vi "ATV Program Global Variables.vi"() -> ()   [LabVIEW 2011]
panel:
  in  "Webcam Data":T1={"Clamp Settings"={"Contrast"=100, "Filter width"=100, "Steepness"=2, "Subsampling Ratio"=1, "Show Search Area"=FALSE, "Show Search Lines"=FALSE, "Show Edges Found"=FALSE, "Show Result"=FALSE}, "Color Plane"=0, "BCG"={"Brightness"=171.0, "Contrast"=55.999992, "Gamma"=2.0}} {"BCG"."Gamma" min=0.1 max=10 step=0.01 scale=10.0..0.1 scale format="%.1f"; "BCG"."Contrast" min=1 max=89 step=0.1 scale=30.0..60.0 scale format="%.2f"; "BCG"."Brightness" min=0 max=255 step=1 scale=0.0..255.0 scale format="%.2f"; "Color Plane" items=["Red", "Green", "Blue", "Hue", "Saturation", "Luminance", "Value", "Intensity"]}
  out "ATV Vision":T2(plugin-control)
  out "Logfile Graph":cluster{dbl[], dbl[]}[](graph)=[{[-121.82428, -121.82428, -121.82428, -121.82428, -121.82428, -121.82428, -121.82428, -121.82428, -121.82428, -121.82428, -121.82428, -121.82428, -121.82428, -121.82428, -121.82428, -121.82428, -121.82428, -121.82428, -121.82428, -121.82428, -121.82428, -121.82428, -121.82428, -121.82428, -121.82428, -121.82428, -121.82428, -121.82428, -121.82428, -121.82428, -121.82428, -121.82428, -121.82428, -121.82428, -121.82428, -121.82428, -121.82428, -121.82428, -121.82428, -121.82428, -121.82428, -121.82428, -121.82428, -121.82428, -121.82428, -121.82428, -121.82428, -121.82428, -121.82428, -121.82428, -121.82428, -121.82428, -121.824573, -121.824573, -121.824573, -121.824573, -121.824573, -121.824573, -121.824573, -121.824573, -121.824573, -121.824573, -121.824573, -121.824573, -121.824573, -121.824573, -121.824573, -121.824573, -121.824573, -121.824573, -121.824573, -121.824573, -121.824573, -121.824573, -121.824573, -121.824573, -121.824573, -121.824573, -121.824573, -121.824573, -121.824573, -121.824573, -121.824573, -121.824573, -121.824573, -121.824573, -121.824573, -121.824573, -121.824573, -121.824573, -121.824573, -121.824573, -121.824573, -121.824573, -121.824573, -121.824573, -121.824573, -121.824573, -121.824573, -121.824573, -121.824573, -121.824573, -121.824573, -121.824573, -121.824573, -121.824573, -121.824573, -121.824573, -121.824573, -121.824573, -121.824573, -121.824573, -121.824573, -121.824573, -121.824573, -121.824573, -121.824573, -121.824573, -121.824573, -121.824573, -121.824573, -121.824573, -121.824573, -121.824573, -121.824573, -121.824573, -121.824573, -121.824573, -121.824573, -121.824373, -121.824373, -121.824373, -121.824373, -121.824373, -121.824373, -121.824373, -121.824373, -121.824373, -121.824373, -121.824373, -121.824373, -121.824373, -121.824373, -121.824373, -121.824373, -121.824373, -121.824373, -121.824373, -121.824373, -121.824373, -121.824373, -121.824373, -121.824373, -121.824373, -121.824373], [39.690327, 39.690327, 39.690327, 39.690327, 39.690327, 39.690327, 39.690327, 39.690327, 39.690327, 39.690327, 39.690327, 39.690327, 39.690327, 39.690327, 39.690327, 39.690327, 39.690327, 39.690327, 39.690327, 39.690327, 39.690327, 39.690327, 39.690327, 39.690327, 39.690327, 39.690327, 39.690327, 39.690327, 39.690327, 39.690327, 39.690327, 39.690327, 39.690327, 39.690327, 39.690327, 39.690327, 39.690327, 39.690327, 39.690327, 39.690327, 39.690327, 39.690327, 39.690327, 39.690327, 39.690327, 39.690327, 39.690327, 39.690327, 39.690327, 39.69047, 39.69047, 39.69047, 39.69047, 39.69047, 39.69047, 39.69047, 39.69047, 39.69047, 39.69047, 39.69047, 39.69047, 39.69047, 39.69047, 39.69047, 39.69047, 39.69047, 39.69047, 39.69047, 39.69047, 39.69047, 39.69047, 39.69047, 39.69047, 39.69047, 39.69047, 39.69047, 39.69047, 39.69047, 39.69047, 39.69047, 39.69047, 39.69047, 39.69047, 39.69047, 39.69047, 39.69047, 39.69047, 39.69047, 39.69047, 39.69047, 39.69047, 39.69047, 39.69047, 39.69047, 39.69047, 39.69047, 39.69047, 39.69047, 39.69047, 39.69047, 39.69047, 39.69047, 39.69047, 39.69047, 39.69047, 39.69047, 39.6908, 39.6908, 39.6908, 39.6908, 39.6908, 39.6908, 39.6908, 39.6908, 39.6908, 39.6908, 39.6908, 39.6908, 39.6908, 39.6908, 39.6908, 39.6908, 39.6908, 39.6908, 39.6908, 39.6908, 39.6908, 39.6908, 39.6908, 39.6908, 39.6908, 39.6908, 39.6908, 39.6908, 39.6908, 39.6908, 39.6908, 39.6905, 39.6905, 39.6905, 39.6905, 39.6905, 39.6905, 39.6905, 39.6905, 39.6905, 39.6905, 39.6905, 39.6905, 39.6905, 39.6905, 39.6905, 39.6905, 39.6905, 39.6905]}, {[-121.824573, -121.824573, -121.824373, -121.824373, -121.824173, -121.824173], [39.69047, 39.6908, 39.6908, 39.6905, 39.6905, 39.69095]}, {[-121.82428, -121.82428, -121.82428, -121.82428, -121.82428, -121.82428, -121.82428, -121.82428, -121.82428, -121.82428, -121.82428, -121.82428, -121.82428, -121.82428, -121.82428, -121.82428, -121.82428, -121.82428, -121.82428, -121.82428, -121.82428, -121.82428, -121.82428, -121.82428, -121.82428, -121.82428, -121.82428, -121.82428, -121.82428, -121.82428, -121.82428, -121.82428, -121.82428, -121.82428, -121.82428, -121.82428, -121.82428, -121.82428, -121.824573, -121.824573, -121.824573, -121.824573, -121.824573, -121.824573, -121.824573, -121.824573, -121.824573, -121.824573, -121.824573, -121.824573, -121.824573, -121.824373, -121.824373, -121.824373, -121.824373, -121.824373, -121.824373, -121.824373, -121.824373, -121.824373, -121.824373, -121.824373, -121.824373, -121.824373, -121.824373, -121.824373, -121.824373, -121.824373, -121.824373, -121.824373, -121.824373, -121.824373, -121.824373, -121.824373, -121.824373, -121.824373, -121.824373], [39.690327, 39.690327, 39.690327, 39.690327, 39.690327, 39.690327, 39.690327, 39.690327, 39.690327, 39.690327, 39.690327, 39.690327, 39.690327, 39.690327, 39.690327, 39.690327, 39.690327, 39.690327, 39.690327, 39.690327, 39.690327, 39.690327, 39.690327, 39.690327, 39.690327, 39.690327, 39.690327, 39.690327, 39.690327, 39.690327, 39.690327, 39.690327, 39.690327, 39.690327, 39.690327, 39.690327, 39.690327, 39.690327, 39.6908, 39.6908, 39.6908, 39.6908, 39.6908, 39.6908, 39.6908, 39.6908, 39.6908, 39.6908, 39.6908, 39.6908, 39.6908, 39.6908, 39.6908, 39.6908, 39.6908, 39.6908, 39.6908, 39.6908, 39.6908, 39.6905, 39.6905, 39.6905, 39.6905, 39.6905, 39.6905, 39.6905, 39.6905, 39.6905, 39.6905, 39.6905, 39.6905, 39.6905, 39.6905, 39.6905, 39.6905, 39.6905, 39.6905]}]
  in  "Map":refnum<k7>(container)
  in  "Map Data":T3={"X"=1000.0, "Y"=1000.0, "Zoom"=19.0, "Map Type"="hybrid", "Google Maps API Key"="AIzaSyDQES5BW68QG5HzTQIG5gxZIUTr_OVHJhg", "Map Refresh Rate (ms)"=5000, "Navigation Path Color"=16860, "Navigation Path Weight"=3, "URL"="http://maps.googleapis.com/maps/api/staticmap?&zoom=13&size=1000x1000&maptype=roadmap&markers=color:blue%7Clabel:S%7C40.702147,-74.015794&markers=color:green%7Clabel:G%7C40.711614,-74.012318&markers=color:red%7Ccolor:red%7Clabel:C%7C40.718217,-73.998284&sensor=false", "Boundary Coordinates"=[{"Latitude"=39.690655, "Longitude"=-121.82408}, {"Latitude"=39.690815, "Longitude"=-121.823863}, {"Latitude"=39.691022, "Longitude"=-121.824048}, {"Latitude"=39.690845, "Longitude"=-121.824595}, {"Latitude"=39.690771, "Longitude"=-121.824607}, {"Latitude"=39.690668, "Longitude"=-121.824669}, {"Latitude"=39.69033, "Longitude"=-121.824234}, {"Latitude"=39.690448, "Longitude"=-121.824055}], "GPS Balloon Character"="1", "Boundary Path Color"=16774656, "Boundary Path Weight"=5, "GPS Balloon Size"="mid", "GPS Balloon Color"="blue", "GPS Path Color"=16711680, "GPS Path Weight"=1, "Disable Google Maps"=FALSE} {"Boundary Coordinates"."Longitude" format="%_12g"; "Boundary Coordinates"."Latitude" format="%_11g"; "Zoom" format="%#.1g"}
  in  "Arduino 2 Data":T4={"Arduino 2 VISA resource"="COM4", "Front Center I2C Data"=[], "Disable Arduino 2"=FALSE, "Rear Left I2C Data"=[], "Rear Right I2C Data"=[]} {"Rear Right I2C Data" format="%x"; "Rear Left I2C Data" format="%x"; "Front Center I2C Data" format="%x"}
  in  "RUN":bool
  in  "Arduino 1 Data":T5={"Arduino 1 VISA resource"="COM6", "Front Right Sonar Analog In Voltage"=5.0, "Front Left Sonar Analog In Voltage"=5.0, "Disable Arduino 1"=FALSE}
  in  "Sonar Data":T6={"Front Left Distance"=0.0, "Front Right Distance"=0.0, "Analog In Filter Rank"=10, "Front Center Distance"=0.0, "Rear Left Distance"=0.0, "Rear Right Distance"=0.0, "Front Left Threshold"=300.0, "Front Right Threshold"=300.0, "Front Center Threshold"=300.0, "Rear Left Threshold"=0.0, "Rear Right Threshold"=0.0}
  in  "Compass Data":cluster{"Angle Uncertainty":dbl, "Heading":dbl}={"Angle Uncertainty"=5.0, "Heading"=0.0}
  in  "Obstacle Avoidance Data":T7={"Obstacle Detected"=FALSE, "Drive Speed"="1", "Steer Angle"="500000", "Left Object"=FALSE, "Right Object"=FALSE, "Center Object"=FALSE, "Rear Left"=FALSE, "Rear Right"=FALSE}
  in  "Navigation Data":T8={"Navigation Coordinates"=[{"Latitude"=39.690557, "Longitude"=-121.824423}, {"Latitude"=39.69085, "Longitude"=-121.824423}, {"Latitude"=39.69085, "Longitude"=-121.824323}, {"Latitude"=39.6904, "Longitude"=-121.824323}, {"Latitude"=39.6904, "Longitude"=-121.824223}, {"Latitude"=39.69095, "Longitude"=-121.824223}, {"Latitude"=39.69095, "Longitude"=-121.824123}, {"Latitude"=39.6907, "Longitude"=-121.824123}, {"Latitude"=39.6907, "Longitude"=-121.824023}, {"Latitude"=39.69095, "Longitude"=-121.824023}], "Coordinate Count"=0, "Drive Speed"="4", "Steer Angle"=450000.0, "Steering"=0.0, "Direction to next Coordinate"=0.0, "Drive"=0.0, "Navigation Path"="Read from File"} {"Drive" scale=0.0..5.0; "Direction to next Coordinate" scale=-180.0..180.0; "Steering" scale=500000.0..-500000.0; "Navigation Coordinates"."Longitude" format="%_12g"; "Navigation Coordinates"."Latitude" format="%_11g"}
  in  "System Data":T9={"End ATV Program"=FALSE, "E-Stop"=FALSE, "Save Logfile"=FALSE, "Logfile Iteration Delay (ms)"=1000, "Loop iteration time (ms)"=100, "Logfile Location"=path "C:/Users/ATV Project/Dropbox/Auto-Steering and Obstacle Avoidance System Project/Software/VI's/_Data/Log_Files(GPS)/GPS_LOG", "Default GPS Navigation Path"=path "C:/Users/ATV Project/Dropbox/Auto-Steering and Obstacle Avoidance System Project/Software/VI's/_Data/GPS_Navigation_Path", "Computer"="ATV", "Default GPS Boundary Path"=path "C:/Users/ATV Project/Dropbox/Auto-Steering and Obstacle Avoidance System Project/Software/VI's/_Data/GPS_Boundary_Path"}
  in  "GPS Data":T10={"GPS VISA resource name"="COM8", "GPS Error"={"status"=FALSE, "code"=0, "source"=""}, "Disable GPS VISA"=FALSE, "Latitude"=39.690327, "Longitude"=-121.82428, "Latitude Uncertainty"=3e-05, "Longitude Uncertainty"=3e-05, "GPS Signal"=0} {"GPS Signal" max=15 step=1 scale=3.0..11.0; "Longitude" format="%_12g"; "Latitude" format="%_11g"}
  in  "Galil Data":T11={"Drive Value Output String"="", "Steer Value Output String"="", "Error Out"={"status"=FALSE, "code"=0, "source"=""}, "Initial Encoder Counts"="0", "Disable Galil Terminal"=FALSE, "Command Input"=""}
  in  "Xbox Data":T12={"Drive Value Output String"="", "Steer Value Output String"="", "Button A"=FALSE, "Button B"=FALSE, "Error Out"={"status"=FALSE, "code"=0, "source"=""}, "Disable XBox Drive & Steer"=FALSE, "Disable XBox Controller"=FALSE, "XBOX Button Trigger Time (ms)"=250, "Button X"=FALSE, "Button Y"=FALSE}
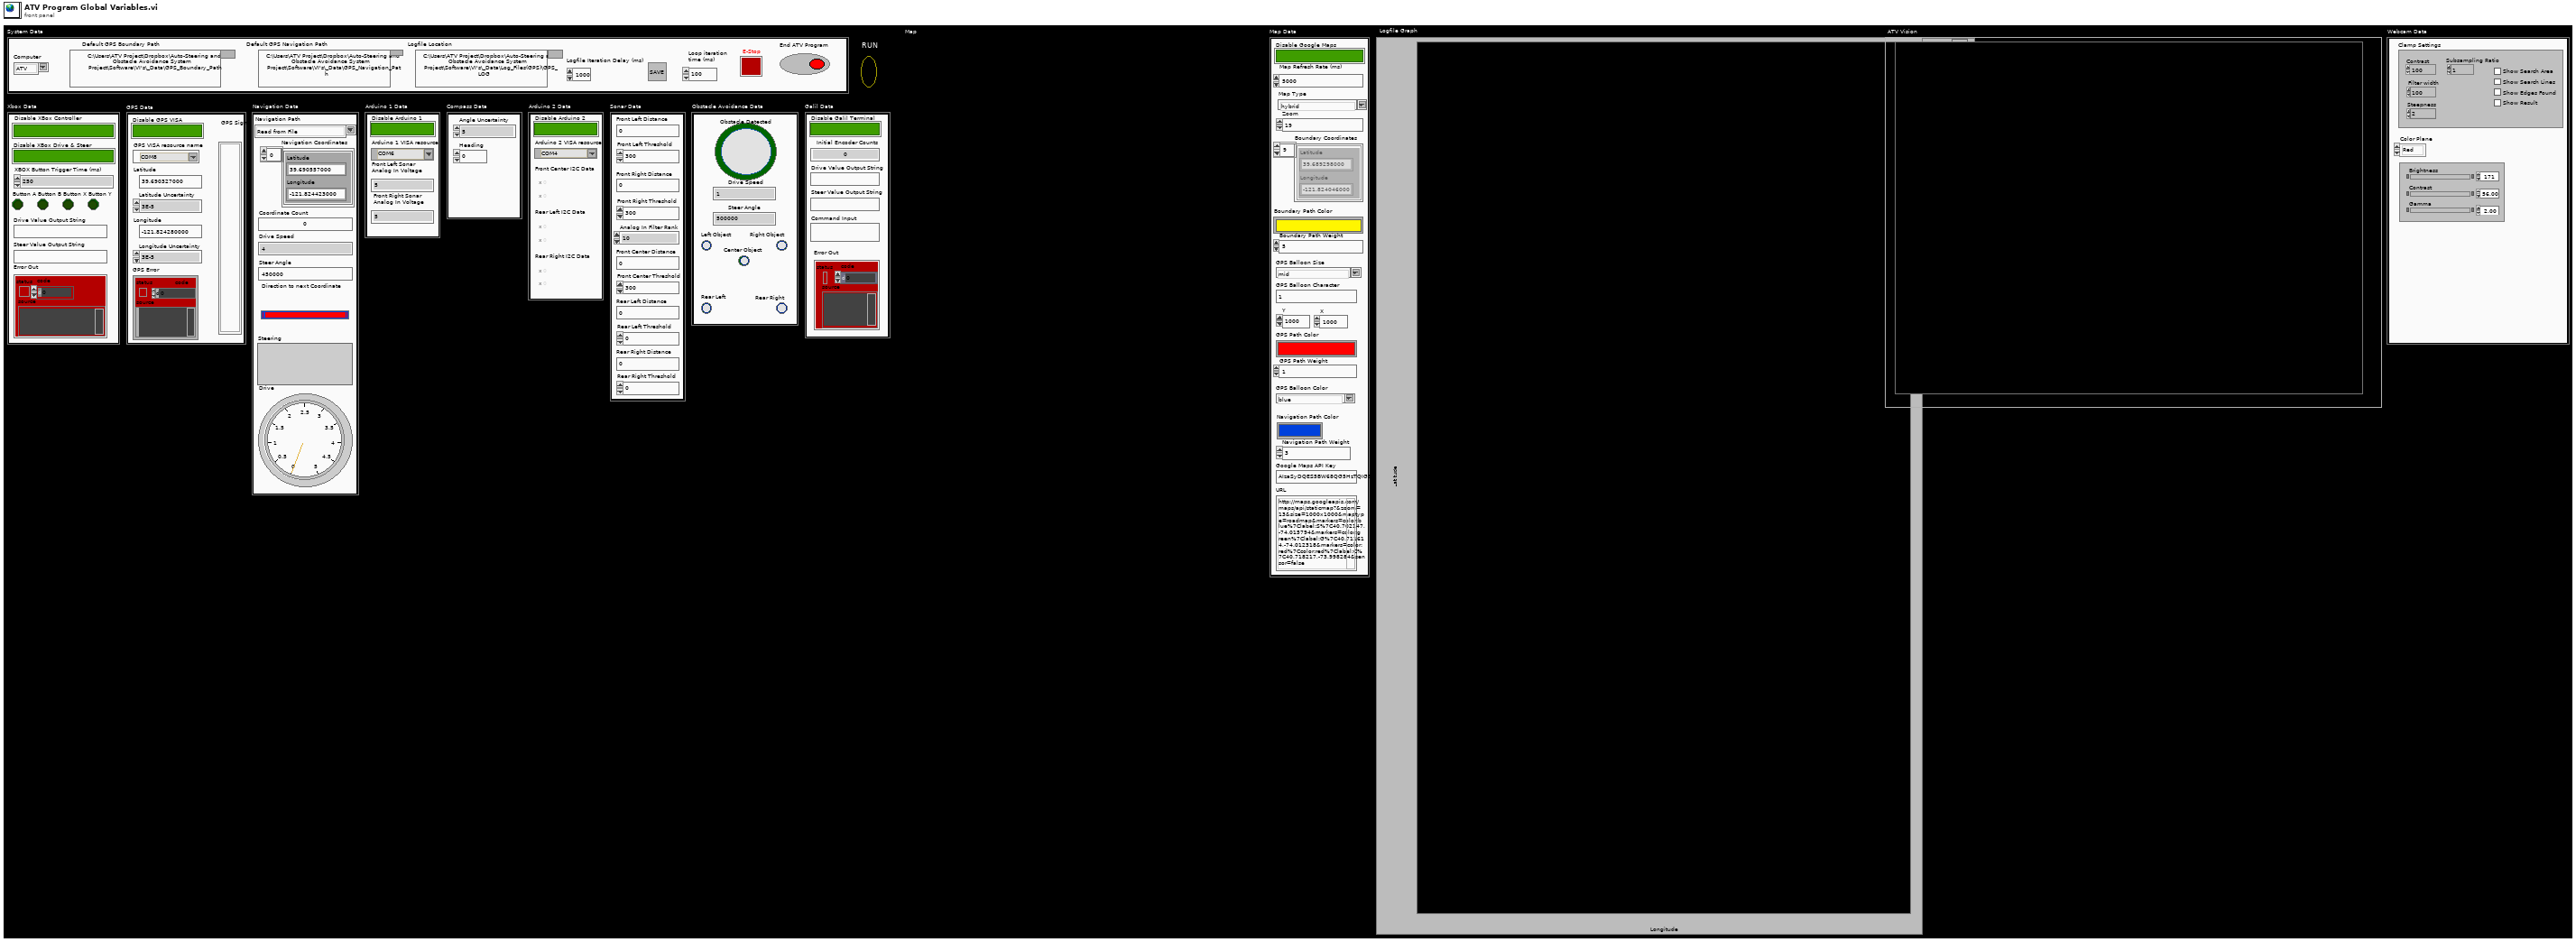
[diagram p1: front panel]
types:
  T1 = cluster{"Clamp Settings":cluster{"Contrast":i32, "Filter width":i32, "Steepness":i32, "Subsampling Ratio":u32, "Show Search Area":bool, "Show Search Lines":bool, "Show Edges Found":bool, "Show Result":bool}, "Color Plane":i32, "BCG":cluster{"Brightness":sgl, "Contrast":sgl, "Gamma":sgl}}
  T2 = typedef "IMAQ Image.ctl" = refnum<image>
  T3 = cluster{"X":dbl, "Y":dbl, "Zoom":sgl, "Map Type":string, "Google Maps API Key":string, "Map Refresh Rate (ms)":u32, "Navigation Path Color":u32, "Navigation Path Weight":i32, "URL":string, "Boundary Coordinates":cluster{"Latitude":dbl, "Longitude":dbl}[], "GPS Balloon Character":string, "Boundary Path Color":u32, "Boundary Path Weight":i32, "GPS Balloon Size":string, "GPS Balloon Color":string, "GPS Path Color":u32, "GPS Path Weight":i32, "Disable Google Maps":bool}
  T4 = cluster{"Arduino 2 VISA resource":refnum<visa-resource-name>, "Front Center I2C Data":u8[], "Disable Arduino 2":bool, "Rear Left I2C Data":u8[], "Rear Right I2C Data":u8[]}
  T5 = cluster{"Arduino 1 VISA resource":refnum<visa-resource-name>, "Front Right Sonar Analog In Voltage":dbl, "Front Left Sonar Analog In Voltage":dbl, "Disable Arduino 1":bool}
  T6 = cluster{"Front Left Distance":dbl, "Front Right Distance":dbl, "Analog In Filter Rank":i32, "Front Center Distance":dbl, "Rear Left Distance":dbl, "Rear Right Distance":dbl, "Front Left Threshold":dbl, "Front Right Threshold":dbl, "Front Center Threshold":dbl, "Rear Left Threshold":dbl, "Rear Right Threshold":dbl}
  T7 = cluster{"Obstacle Detected":bool, "Drive Speed":string, "Steer Angle":string, "Left Object":bool, "Right Object":bool, "Center Object":bool, "Rear Left":bool, "Rear Right":bool}
  T8 = cluster{"Navigation Coordinates":cluster{"Latitude":dbl, "Longitude":dbl}[], "Coordinate Count":u32, "Drive Speed":string, "Steer Angle":dbl, "Steering":dbl, "Direction to next Coordinate":dbl, "Drive":dbl, "Navigation Path":string}
  T9 = cluster{"End ATV Program":bool, "E-Stop":bool, "Save Logfile":bool, "Logfile Iteration Delay (ms)":u32, "Loop iteration time (ms)":u32, "Logfile Location":path, "Default GPS Navigation Path":path, "Computer":string, "Default GPS Boundary Path":path}
  T10 = cluster{"GPS VISA resource name":refnum<visa-resource-name>, "GPS Error":errorcluster, "Disable GPS VISA":bool, "Latitude":dbl, "Longitude":dbl, "Latitude Uncertainty":dbl, "Longitude Uncertainty":dbl, "GPS Signal":u32}
  T11 = cluster{"Drive Value Output String":string, "Steer Value Output String":string, "Error Out":errorcluster, "Initial Encoder Counts":string, "Disable Galil Terminal":bool, "Command Input":string}
  T12 = cluster{"Drive Value Output String":string, "Steer Value Output String":string, "Button A":bool, "Button B":bool, "Error Out":errorcluster, "Disable XBox Drive & Steer":bool, "Disable XBox Controller":bool, "XBOX Button Trigger Time (ms)":u32, "Button X":bool, "Button Y":bool}
diagram:
